vi "PCAN_CompMessage.vi"(7 "Excitation":bool, 8 "Detector4":bool, 9 "Detector3":bool, 10 "Detector2":bool, 11 "Detector1":bool) -> (1 "CAN_Message":T1)   [LabVIEW 2010]
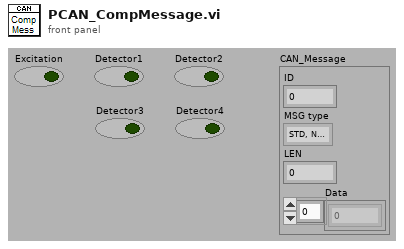
[diagram p1: front panel]
types:
  T1 = cluster{"ID":u32, "MSG type":enum8{"STD, NO RTR", "STD,RTR", "XTD, NO RTR", "XTD, RTR"}, "LEN":u8, "Data":u8[]}
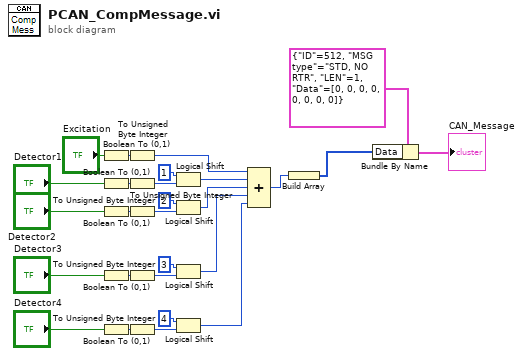
[diagram p0: block diagram]
diagram:
  n1 = Boolean To (0,1)(Boolean="Excitation") -> (0, 1=w14:i16)
  n2 = Boolean To (0,1)(Boolean="Detector1") -> (0, 1=w15:i16)
  n3 = Boolean To (0,1)(Boolean="Detector2") -> (0, 1=w17:i16)
  n4 = Boolean To (0,1)(Boolean="Detector3") -> (0, 1=w9:i16)
  n5 = Boolean To (0,1)(Boolean="Detector4") -> (0, 1=w7:i16)
  n6 = To Unsigned Byte Integer(number=w14) -> (unsigned 8bit integer=w25:u8)
  n7 = To Unsigned Byte Integer(number=w15) -> (unsigned 8bit integer=w19:u8)
  n8 = To Unsigned Byte Integer(number=w17) -> (unsigned 8bit integer=w21:u8)
  n9 = To Unsigned Byte Integer(number=w9) -> (unsigned 8bit integer=w10:u8)
  n10 = To Unsigned Byte Integer(number=w7) -> (unsigned 8bit integer=w8:u8)
  n11 = Logical Shift(y=i8 1, x=w19) -> (x << y=w23:u8)
  n12 = Logical Shift(y=i8 2, x=w21) -> (x << y=w24:u8)
  n13 = Logical Shift(y=i8 3, x=w10) -> (x << y=w6:u8)
  n14 = Logical Shift(y=i8 4, x=w8) -> (x << y=w5:u8)
  n15 = Compound Arithmetic op=ADD(w25, w23, w24, w6, w5) -> (w26:u8)
  n16 = Build Array(w26) -> (w27:u8[])
  n17 = Bundle By Name(cluster=T1 {"ID"=512, "MSG type"=enum."STD, NO RTR", "LEN"=1, "Data"=[0, 0, 0, 0, 0, 0, 0, 0]} ("CAN_Message"), "Data"=w27) -> (→"CAN_Message":T1)
